vi "Start.vi"(8 "error in (no error)":errorcluster, 11 "DAQmx Base CFG in":refnum<class "DAQmx Base CFG.lvclass">) -> (0 "error out":errorcluster, 3 "DAQmx Base CFG out":refnum<class "DAQmx Base CFG.lvclass">)   [LabVIEW 2023, in "DAQmx Base CFG.lvclass"]
uses:
  DAQmx Base CFG.lvclass
  DAQmx Base CFG.lvclass/DAQmx Base CFG.ctl
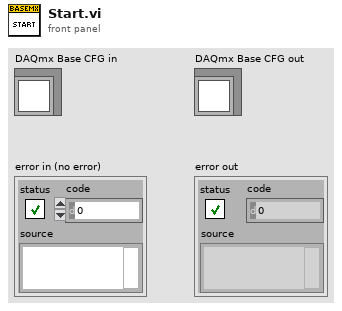
[diagram p1: front panel]
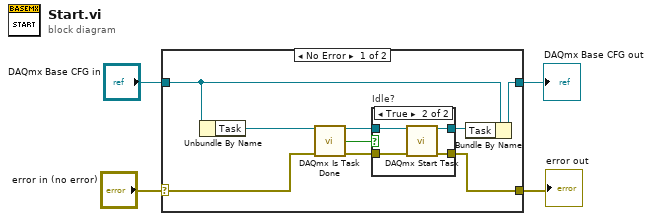
[diagram p0: block diagram]
diagram:
  n1 = case shown="No Error" "error in (no error)" {
    selector: "error in (no error)" -> [w13 w21]
    tunnel: "DAQmx Base CFG in" -> [w11 w20]
    tunnel: [w10 w20] -> w1
    tunnel: [w12 w21] -> w2
    frame No Error {
      n2 = Unbundle By Name(w11) -> ("Task"=w7:refnum<k21>)
      n3 = call <vilib>:"DAQmx Is Task Done.vi"("task/channels in"=w7, "error in"=w13) -> ("task out"=w6:refnum<k21>, "task done?"=w5:bool, "error out"=w8:errorcluster)  [unwired: 11 in]
      n4 = case "Idle?" shown="True" w5 {
        tunnel: [w15 w19] -> w12
        tunnel: [w14 w18] -> w9
        tunnel: w8 -> [w15 w17]
        tunnel: w6 -> [w14 w16]
        frame False {
        }
        frame True {
          n5 = call <vilib>:"DAQmx Start Task.vi"("task/channels in"=w16, "error in"=w17) -> ("task out"=w18:refnum<k21>, "error out"=w19:errorcluster)  [unwired: 12 in]
        }
      }
      n6 = Bundle By Name(cluster=w11, "Task"=w9) -> (w10:refnum<class "DAQmx Base CFG.lvclass">)
    }
    frame Error {
    }
  }
  "error out" <- w2
  "DAQmx Base CFG out" <- w1
